vi "Servos.vi"(2 "ServosWarmHigh (us)KaltHigh(us)":T1, 3 "ServoTrap2kalt":bool, 4 "ServoTrap1kalt":bool) -> ()   [LabVIEW 2010]
uses:
  <vilib>/eio/EIONode/EIONode.xnode
  <vilib>/rvi/eio/nirviEIOImplementation/nirviEIOImplementation.xnode
  <vilib>/rvi/eio/common/nirviEmuClasses.ctl
  <vilib>/rvi/eio/common/nirviEmuTemplateMethod_noerrors.vi
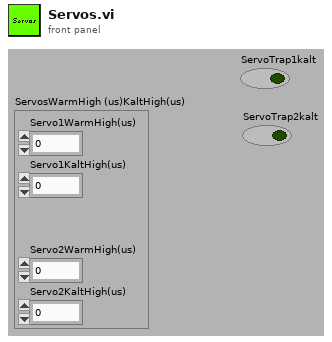
[diagram p1: front panel]
types:
  T1 = cluster{"Servo1WarmHigh(us)":u32, "Servo1KaltHigh(us)":u32, "Servo2WarmHigh(us)":u32, "Servo2KaltHigh(us)":u32}
  T2 = typedef "nirviEmuClasses.ctl" = enum16{"IO Read", "IO Write", "Method", "Property Read", "Property Write"}
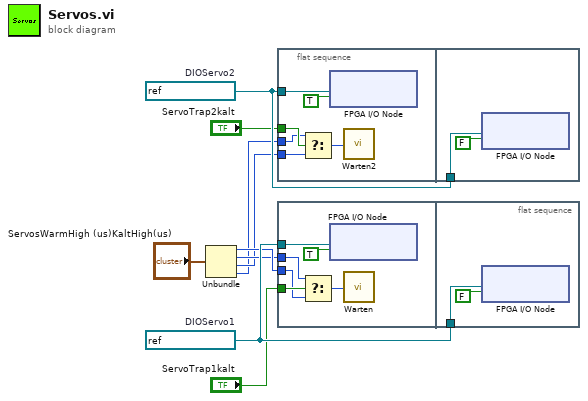
[diagram p0: block diagram]
diagram:
  w9 = refnum<k21> "Mod6/DIO3"  # DIOServo2
  w8 = refnum<k21> "Mod6/DIO2"  # DIOServo1
  n1 = Unbundle("ServosWarmHigh (us)KaltHigh(us)") -> ("Servo1WarmHigh(us)"=w6:u32, "Servo1KaltHigh(us)"=w5:u32, "Servo2WarmHigh(us)"=w4:u32, "Servo2KaltHigh(us)"=w3:u32)
  n2 = flat-sequence {
    tunnel: w9 -> [w15]
    tunnel: "ServoTrap2kalt" -> [w13]
    tunnel: w3 -> [w12]
    tunnel: w4 -> [w11]
    tunnel: w9 -> [w28]
    frame #0 {
      n3 = Select(t=w12, s=w13, f=w11) -> (s? t:f=w10:u32)
      n4 = xnode "FPGA I/O Node"("I/O Item"=TRUE, "FPGA I/O In"=w15) -> ()  [unwired: 1 out]
      n5 = call "Warten2"("Count(uSec)"=w10) -> ()  [unwired: 1 out]
    }
    frame #1 {
      n6 = xnode "FPGA I/O Node"("I/O Item"=FALSE, "FPGA I/O In"=w28) -> ()  [unwired: 1 out]
    }
  }
  n7 = flat-sequence {
    tunnel: w8 -> [w45]
    tunnel: "ServoTrap1kalt" -> [w43]
    tunnel: w5 -> [w42]
    tunnel: w6 -> [w41]
    tunnel: w8 -> [w58]
    frame #0 {
      n8 = Select(t=w42, s=w43, f=w41) -> (s? t:f=w40:u32)
      n9 = xnode "FPGA I/O Node"("I/O Item"=TRUE, "FPGA I/O In"=w45) -> ()  [unwired: 1 out]
      n10 = call "Warten"("Count(uSec)"=w40) -> ()  [unwired: 1 out]
    }
    frame #1 {
      n11 = xnode "FPGA I/O Node"("I/O Item"=FALSE, "FPGA I/O In"=w58) -> ()  [unwired: 1 out]
    }
  }
